vi "COMTRADE Write Private Inf.vi"   [LabVIEW 2012, in "NI_EP_COMTRADE.lvlib"]
doc: "Writes data to the private sections of the optionally specified .inf file. If the <B>entry name</B> you specify already exists, this VI replaces the existing entry. You must set <B>include information file?</B> to TRUE in the COMTRADE Open VI to open the .inf file. Otherwise this VI returns an error."
uses:
  <vilib>/addons/Electrical Power/File IO/NI_EP_COMTRADE.lvlib
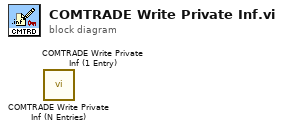
[diagram p0: block diagram]
diagram:
  n1 = call <vilib>:"COMTRADE Write Private Inf (N Entries).vi"() -> ()  [unwired: 8 in, 4 out]
  n2 = call <vilib>:"COMTRADE Write Private Inf (1 Entry).vi"() -> ()  [unwired: 8 in, 4 out]
